vi "DSF.Engine.Status.Framework.Performance.Set Rx Duration.vi"(8 "error in (no error)":errorcluster, 10 "rx duration":u32 format="%d us", 11 "Framework Performance in":refnum<class "DSF.Engine.Status.Framework.Performance.lvclass">) -> (0 "error out":errorcluster, 3 "Framework Performance out":refnum<class "DSF.Engine.Status.Framework.Performance.lvclass">)   [LabVIEW 2017, in "Data Sharing Framework Engine.lvlib" / "DSF.Engine.Status.Framework.Performance.lvclass"]
uses:
  DSF.Engine.Status.Framework.Performance.lvclass
  DSF.Engine.Status.Framework.Performance.lvclass/DSF.Engine.Status.Framework.Performance.ctl
  <vilib>/National Instruments/Memory Manager/Classes/Pointer/Memory.Pointer.lvclass/Memory.Pointer.ctl
  <vilib>/National Instruments/Memory Manager/Classes/Pointer/Memory.Pointer.Write.0D.U32.vi
  <vilib>/National Instruments/Memory Manager/Classes/Pointer/Memory.Pointer.Write.No Check.0D.U32.vi
  <vilib>/National Instruments/Memory Manager/Classes/Pointer/Memory.Pointer.Parameter Check.Null Pointer.vi
  <vilib>/National Instruments/Memory Manager/Classes/Pointer/Memory.Pointer.Parameter Check.Subset.vi
  <vilib>/National Instruments/Memory Manager/Classes/Pointer/Memory.Pointer.Get Address.vi
  <vilib>/National Instruments/Memory Manager/Classes/Pointer/Memory.Pointer.Errors.vi
  <vilib>/National Instruments/Memory Manager/Classes/Pointer/Memory.Pointer.Errors.Null Pointer.vi
  <vilib>/National Instruments/Memory Manager/Classes/Pointer/Memory.Pointer.Errors.Out of Bounds.vi
  <vilib>/National Instruments/Memory Manager/Classes/Pointer/Memory.Pointer.Get Size.vi
  <vilib>/National Instruments/Memory Manager/Classes/Pointer/Memory.Pointer.Errors.Create Error.vi
  <vilib>/NI/Static Error Handling/VIs/Static Error Handling.Source Buffer.Write.String.vi
  <vilib>/National Instruments/Memory Manager/Classes/Pointer/Memory.Pointer.Errors.Write Pointer Size.vi
  <vilib>/NI/Static Error Handling/VIs/Static Error Handling.Source Buffer.Write.Numeric.Scalar.Base10.vi
  <vilib>/NI/Static Error Handling/VIs/Static Error Handling.Source Buffer.Write.Numeric.Scalar.Base10 (U64).vi
  <vilib>/NI/Static Error Handling/VIs/Static Error Handling.Error Cluster Constant.vi
  <vilib>/NI/Static Error Handling/VIs/Static Error Handling.Error Cluster Constant (512B).vi
  <vilib>/NI/Static Error Handling/VIs/Static Error Handling.Parameters.Status.Set.vi
  <vilib>/NI/Static Error Handling/VIs/Static Error Handling.Parameters.Code.Set.vi
  <vilib>/NI/Static Error Handling/VIs/Static Error Handling.Parameters.VI Source.Set.vi
  <vilib>/National Instruments/Memory Manager/Constants/Memory.Constants.vi
  <vilib>/National Instruments/Memory Manager/Constants/Memory.Constants.Library Name.vi
  <vilib>/National Instruments/Memory Manager/Classes/Pointer/Memory.Pointer.Errors.Get Info.vi
  <vilib>/National Instruments/Memory Manager/Classes/Pointer/Memory.Pointer.lvclass
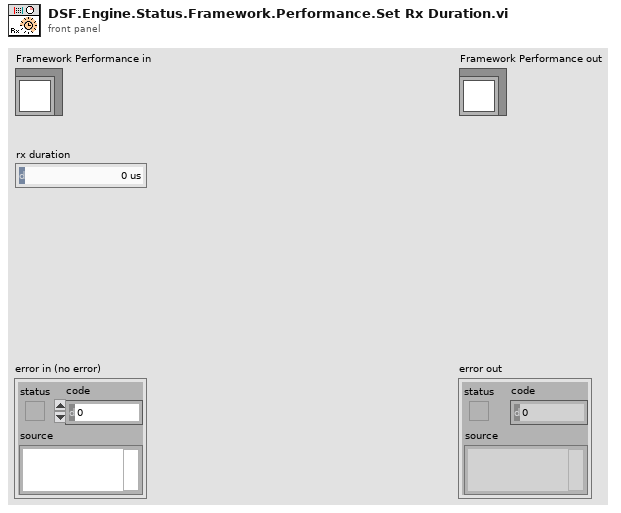
[diagram p1: front panel]
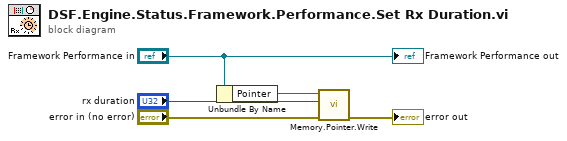
[diagram p0: block diagram]
diagram:
  n1 = Unbundle By Name("Framework Performance in") -> ("Pointer"=w5:refnum<class "Memory.Pointer.lvclass">)
  n2 = call-poly <vilib>:"Memory.Pointer.Write.vi"("error in (no error)"="error in (no error)", "value"="rx duration", "Pointer in"=w5) -> ("error out"=→"error out":errorcluster)  [unwired: 5 in, 3 out]
  "Framework Performance out" <- "Framework Performance in"
